vi "Lvi Write Dbl Data1D.vi"(7 "NumSamples":u32, 8 "error in (no error)":errorcluster, 9 "DataBuf":dbl[](array[numeric])=array[4097 elements], 10 "timeout":dbl, 11 "TaskRef":i32) -> (0 "error out":errorcluster, 1 "NumQueued out":u32, 2 "function return":u32(ring), 3 "TaskRef out":i32)   [LabVIEW 2022 SP3, in "DtLvLink.lvlib"]
doc: "Calls directly into the entry points of the DLL of the Data Acq SDK to write a one-dimensional array of double data points to the virtual channels of a task you specify. This VI is used by the higher-level VI, DtOLWrite."
uses:
  DtLvLink.lvlib
  <userlib>/LV-Link3/DtLvLink_64.dll
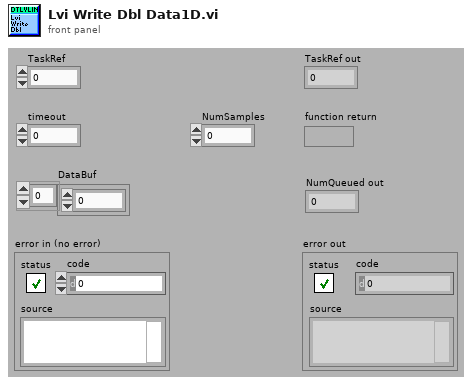
[diagram p1: front panel]
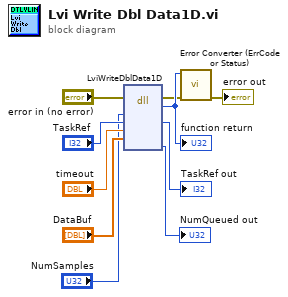
[diagram p0: block diagram]
diagram:
  n1 = dll-call lib="C:/Program Files/National Instruments/LabVIEW 2022/user.lib/LV-Link3/DtLvLink_64.*" fn="LviWriteDblData1D"(error in="error in (no error)", "NumSamples"="NumSamples", "TaskRef"="TaskRef", "timeout"="timeout", "DataBuf"="DataBuf") -> (error out=w3:errorcluster, "return type"=w10:u32, "TaskRef"=→"TaskRef out":i32, "NumQueued"=→"NumQueued out":u32)  [unwired: 6 in, 1 out]
  "function return" <- w10
  n2 = call "Error Converter (ErrCode or Status).vi"("error in (no error)"=w3, "error code"=w10) -> ("error out"=→"error out":errorcluster)  [unwired: 9 in]
